vi "Do.vi"(8 "error in (no error)":errorcluster, 10 "Actor in":refnum<class "Actor.lvclass">, 11 "Handle Drop Msg":refnum<class "Handle Drop Msg.lvclass">) -> (0 "error out":errorcluster, 2 "Actor out":refnum<class "Actor.lvclass">)   [LabVIEW 2017, in "Handle Drop Msg.lvclass"]
doc: "This VI delivers the message to the actor by calling the appropriate method(s) on the actor."
uses:
  <vilib>/gpm_packages/@cs/Test-executive-builder/Source/Test Executive Builder View/Test Executive Builder View Messages/Handle Drop Msg/Handle Drop Msg.lvclass
  <vilib>/ActorFramework/Actor/Actor.lvclass
  <vilib>/gpm_packages/@cs/Test-executive-builder/Source/Test Executive Builder View/Test Executive Builder View/Test Executive Builder View.lvclass
  C:/Program Files/National Instruments/LabVIEW 2017/vi.lib/ActorFramework/Actor/Actor.lvclass
  <vilib>/gpm_packages/@cs/Test-executive-builder/Source/Test Executive Builder View/Test Executive Builder View Messages/Handle Drop Msg/Handle Drop Msg.lvclass/Handle Drop Msg.ctl
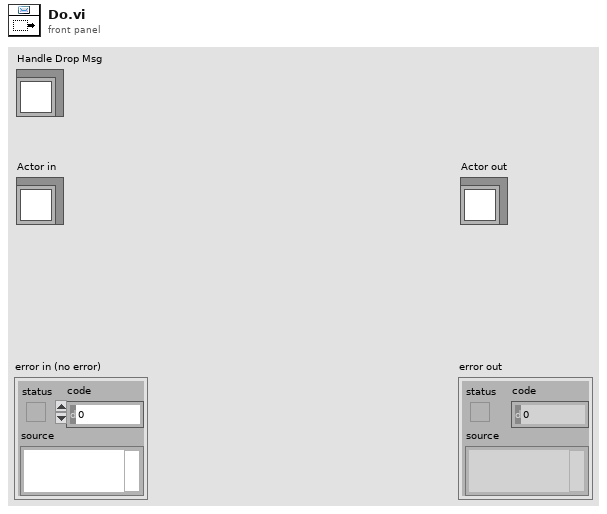
[diagram p1: front panel]
types:
  T1 = typedef "LVPoint32TypeDef.ctl" = cluster{"Horizontal":i32, "Vertical":i32}
  T2 = cluster{"Shift":bool, "Ctrl":bool, "Alt":bool, "Cmd":bool, "Opt":bool}
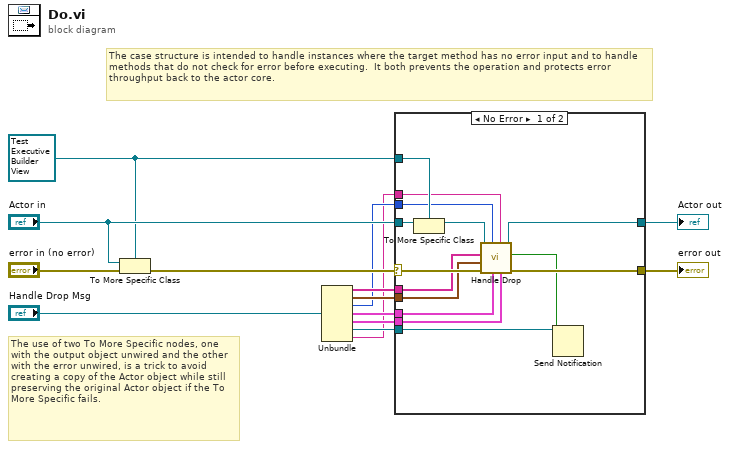
[diagram p0: block diagram]
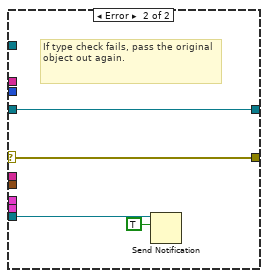
[diagram p2: hidden frame]
diagram:
  w8 = refnum<class "Test Executive Builder View.lvclass"> refnum ("Actor in")
  # "The use of two To More Specific nodes, one with the output object unwired and the other with the error unwired, is a trick to avoid creating a copy of the Actor object while still preserving the original Actor object if the To More Specific fails."
  # "The case structure is intended to handle instances where the target method has no error input and to handle methods that do not check for error before executing.  It both prevents the operation and protects error throughput back to the actor core."
  n1 = To More Specific Class(target class=w8, reference="Actor in", error in="error in (no error)") -> (error out=w12:errorcluster)  [unwired: 1 out]
  n2 = Unbundle("Handle Drop Msg") -> (w7:string[], w6:T1, w5:u16, w4:T2, w3:cluster{"Double Click":bool, "Menu Key":bool}, w2:refnum<notifier>, w1:string)
  n3 = case shown="No Error" w12 {
    selector: w12 -> [w26 w32]
    tunnel: [w28 w32] -> w11
    tunnel: [w27 w31] -> w10
    tunnel: "Actor in" -> [w25 w31]
    tunnel: w8 -> [w24 _]
    tunnel: w7 -> [w22 _]
    tunnel: w6 -> [w21 _]
    tunnel: w5 -> [w20 _]
    tunnel: w4 -> [w19 _]
    tunnel: w3 -> [w18 _]
    tunnel: w2 -> [w17 w30]
    tunnel: w1 -> [w15 _]
    frame No Error {
      n4 = To More Specific Class(target class=w24, reference=w25) -> (specific class reference=w23:refnum<class "Test Executive Builder View.lvclass">)  [unwired: 1 in, 1 out]
      n5 = call-dynamic "Handle Drop.vi"("Mods"=w18, "Tag"=w15, "PlatMods"=w19, "Button"=w20, "error in (no error)"=w26, "Coords"=w21, "Available Data Names"=w22, "Test Executive Builder View in"=w23) -> ("error out"=w28:errorcluster, "Discard?"=w16:bool, "Test Executive Builder View out"=w27:refnum<class "Test Executive Builder View.lvclass">)  [unwired: 1 in]
      n6 = Send Notification(notification=w16, notifier=w17) -> ()  [unwired: 1 in, 2 out]
    }
    frame Error {
      # "If type check fails, pass the original object out again."
      n7 = Send Notification(notification=TRUE, notifier=w30) -> ()  [unwired: 1 in, 2 out]
    }
  }
  "error out" <- w11
  "Actor out" <- w10
